vi "Simple Send UI Manipulation CMD.vi"(4 "Any Data 2":variant, 6 "Any Data":variant, 8 "error in (no error)":errorcluster, 9 "UI Manipulation CMD":i64, 10 "Smiple UI Console ID":i64, 11 "UI Console in":refnum<class "UI Console.lvclass">) -> (0 "error out":errorcluster, 3 "UI Console out":refnum<class "UI Console.lvclass">)   [LabVIEW 2024, in "UI Console.lvclass"]
uses:
  UI Console.lvclass
  UI Console MSG/UI Console MSG.lvclass
  Ancestor Class/Message/Type Def/CMD Type.ctl
  UI Console MSG/Type Def/UI Console 1st CMD.ctl
  Ancestor Class/Message/Message.lvclass/Message.ctl
  UI Console MSG/UI Console MSG.lvclass/UI Console MSG.ctl
  Ancestor Class/Message/Public Data/Write CMD Type.vi
  UI Console MSG/Public Data/Write UI Console 1st CMD.vi
  UI Console MSG/Public Data/Write UI Manipulation CMD.vi
  Ancestor Class/Message/Public Data/Write Any Data.vi
  Ancestor Class/Message/Write Any Data 2.vi
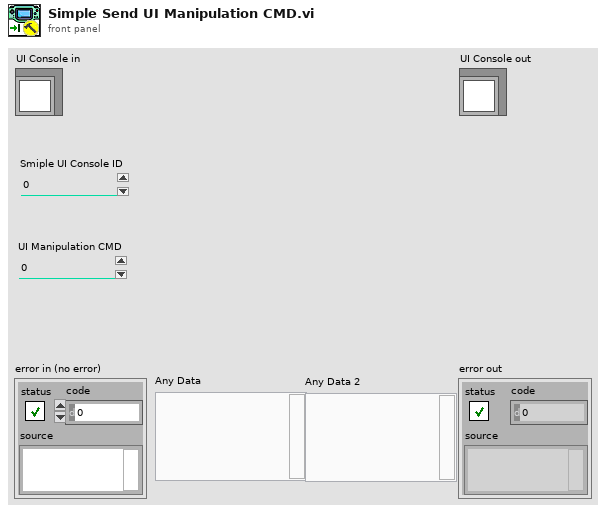
[diagram p1: front panel]
types:
  T1 = typedef "UI Console 1st CMD.ctl" = enum16{"None", "UI Manipulation", "UI Operation", "UI Stop"}
  T2 = typedef "CMD Type.ctl" = enum16{"None", "General CMD", "1st CMD", "2nd CMD", "3rd CMD", "4th CMD", "5th CMD", "6th CMD", "7th CMD"}
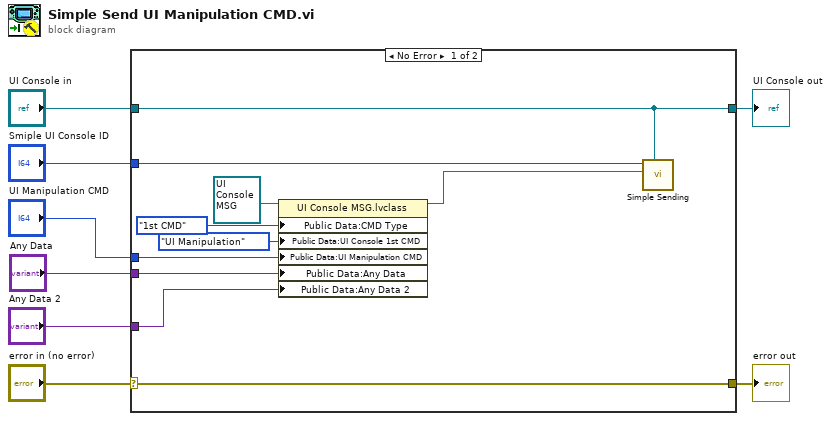
[diagram p0: block diagram]
diagram:
  n1 = case shown="No Error" "error in (no error)" {
    selector: "error in (no error)" -> [w18 w20]
    tunnel: [w18 w20] -> w7
    tunnel: [w17 w19] -> w5
    tunnel: "UI Console in" -> [w17 w19]
    tunnel: "Smiple UI Console ID" -> [w16 _]
    tunnel: "UI Manipulation CMD" -> [w12 _]
    tunnel: "Any Data" -> [w11 _]
    tunnel: "Any Data 2" -> [w10 _]
    frame No Error {
      n2 = property class="UI Console MSG.lvclass"(reference=refnum<class "UI Console MSG.lvclass"> refnum ("UI Console MSG.lvclass"), "Public Data:CMD Type"=CMD_Type."1st CMD" ("CMD Type"), "Public Data:UI Console 1st CMD"=UI_Console_1st_CMD."UI Manipulation" ("UI Console 1st CMD"), "Public Data:UI Manipulation CMD"=w12, "Public Data:Any Data"=w11, "Public Data:Any Data 2"=w10) -> (reference out=w9:refnum<class "UI Console MSG.lvclass">)  [unwired: 1 in, 1 out]
      n3 = call "Simple Sending.vi"("System Actor In"=w17, "Message In"=w9, "ID In"=w16) -> ()  [unwired: 9 in]
    }
    frame Error {
    }
  }
  "error out" <- w7
  "UI Console out" <- w5
